vi "test_VISAFactory_InitializeMeasurementLinkSessionWithAttachAndDetach_RemoteSessionAttachedAndDetached.vi"(8 "error in":errorcluster) -> (0 "error out":errorcluster, 2 "result":string, 3 "pass":bool)   [LabVIEW 2020, in "MeasurementServerTests.lvlib"]
uses:
  MeasurementServerTests.lvlib
  Runtime/Sessions/Instrument Sessions/ISession Factory/Initialize and Close Session Behavior.ctl
  Runtime/Sessions/Instrument Sessions/ISession Factory/ISession Factory.lvclass
  Runtime/Sessions/VISA Sessions/Session Factory/Session Factory.lvclass
  <vilib>/Instr/_visa.llb/VISA Open Access Mode.ctl
  <vilib>/NI-VISA/VISA gRPC Open Close Behavior.ctl
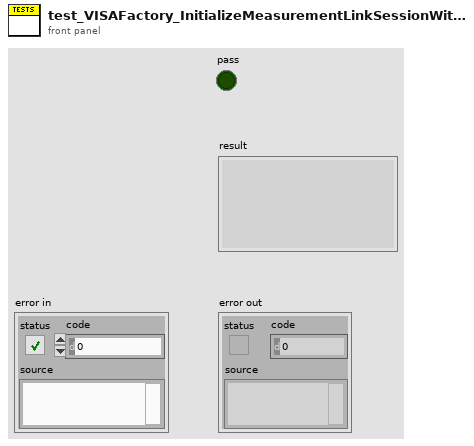
[diagram p1: front panel]
types:
  T1 = typedef "VISA gRPC Open Close Behavior.ctl" = enum16{"Auto", "Initialize and Close", "Attach and Detach", "Initialize and Detach", "Attach and Close"}
  T2 = typedef "VISA Open Access Mode.ctl" = u32
  T3 = typedef "Plug-In SDK Instrument Sessions.lvlib/ISession Factory.lvclass/Remote Connection Options.ctl" = cluster{"session name":string, "address":string, "port":u32}
  T4 = typedef "Plug-In SDK Instrument Sessions.lvlib/ISession Factory.lvclass/Initialize and Close Session Behavior.ctl" = enum16{"Initialize and Close", "Attach and Detach", "Initialize and Detach", "Attach and Close"}
  T5 = typedef "Plug-In SDK Instrument Sessions.lvlib/ISession Factory.lvclass/Session Initialization Parameters.ctl" = cluster{"resource name":string, "session name":string}
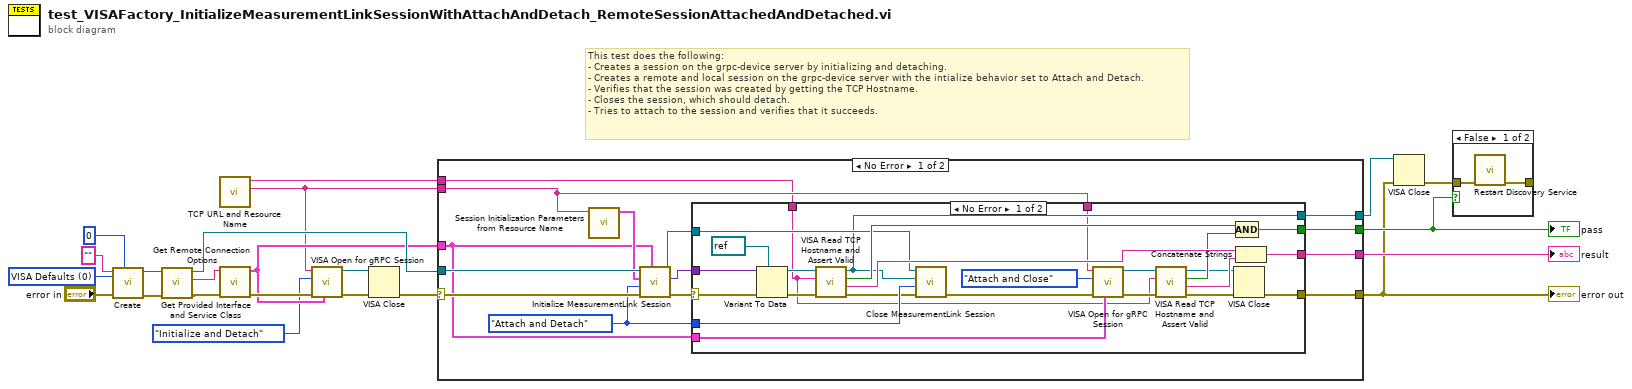
[diagram p0: block diagram]
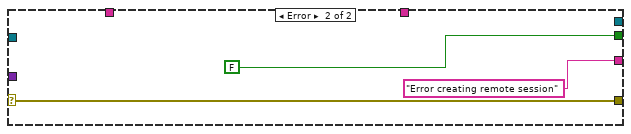
[diagram p2: hidden frame]
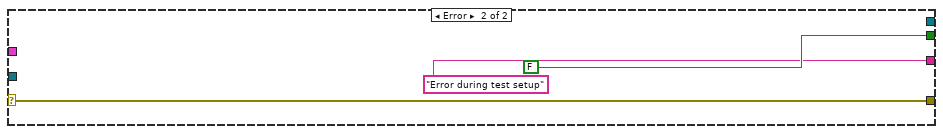
[diagram p3: hidden frame]
diagram:
  w9 = T2 0 items=["VISA Defaults"=0, "Exclusive Lock"=1, "Load Configured Settings"=4] ("access mode")
  # "This test does the following:\n- Creates a session on the grpc-device server by initializing and detaching.\n- Creates a remote and local session on the grpc-device server with the intialize behavior set to Attach and Detach.\n- Verifies that the session was created by getting the TCP Hostname.\n- Closes the session, which should detach.\n- Tries to attach to the session and verifies that it succeeds."
  n1 = call "Create.vi"("visa open timeout"=u32 0, "error in"="error in", "access mode"=w9, "instrument type id"="") -> ("error out"=w14:errorcluster, "session factory out"=w13:refnum<class "Session Factory.lvclass">)  [unwired: 6 in]
  n2 = call-dynamic "Get Provided Interface and Service Class.vi"("error in"=w14, "session factory in"=w13) -> ("error out"=w15:errorcluster, "provided interface"=w12:string, "session factory out"=w16:refnum<class "Session Factory.lvclass">)  [unwired: 6 in, 1 out]
  n3 = call "TCP URL and Resource Name.vi"() -> ("visa resource name"=w2:string, "url"=w1:string)  [unwired: 10 in]
  n4 = call "Get Remote Connection Options.vi"("error in"=w15, "provided interface"=w12) -> ("error out"=w8:errorcluster, "remote connection options"=w7:T3)  [unwired: 8 in]
  n5 = call <vilib>:"VISA Open for gRPC Session.vi"("gRPC Options"=w7, "error in (no error)"=w8, "open/close behavior"=VISA_gRPC_Open_Close_Behavior."Initialize and Detach" ("Open/Close Behavior"), "VISA resource name"=w2) -> ("error out"=w4:errorcluster, "VISA resource name out"=w3:refnum<visa-resource-name>)  [unwired: 6 in]
  n6 = VISA Close(VISA resource name=w3, error in (no error)=w4) -> (error out=w5:errorcluster)
  n7 = case shown="No Error" w5 {
    selector: w5 -> [w31 w65]
    tunnel: [w35 w65] -> w18
    tunnel: [w36 FALSE] -> w19
    tunnel: [w34 "Error during test setup" ("f")] -> w22
    tunnel: w7 -> [w25 _]
    tunnel: w16 -> [w30 _]
    tunnel: [w29 _] -> w21
    tunnel: w2 -> [w24 _]
    tunnel: w1 -> [w23 _]
    frame No Error {
      w26 = Initialize_and_Close_Session_Behavior."Attach and Detach" ("initialize and close session behavior")
      n8 = call "Session Initialization Parameters from Resource Name.vi"("resource name"=w24) -> ("session initialization parameters"=w28:T5)  [unwired: 10 in]
      n9 = call-dynamic "Initialize MeasurementLink Session.vi"("remote connection options"=w25, "error in"=w31, "initialize and close session behavior"=w26, "session initialization parameters"=w28, "session factory in"=w30) -> ("error out"=w32:errorcluster, "session out"=w33:variant, "session factory out"=w27:refnum<class "Session Factory.lvclass">)  [unwired: 4 in]
      n10 = case shown="No Error" w32 {
        selector: w32 -> [w60 w63]
        tunnel: [w56 FALSE] -> w36
        tunnel: [w46 w63] -> w35
        tunnel: [w54 "Error creating remote session"] -> w34
        tunnel: w33 -> [w61 _]
        tunnel: [w51 _] -> w29
        tunnel: w27 -> [w52 _]
        tunnel: w26 -> [w50 _]
        tunnel: w24 -> [w48 _]
        tunnel: w25 -> [w45 _]
        tunnel: w23 -> [w37 _]
        frame No Error {
          n11 = Variant To Data(error in=w60, type=refnum<visa-resource-name> refnum ("VISA resource name out"), Variant=w61) -> (data=w57:refnum<visa-resource-name>, error out=w58:errorcluster)
          n12 = call "VISA Read TCP Hostname and Assert Valid.vi"("error in"=w58, "expected hostname"=w37, "visa refnum in"=w57) -> ("error out"=w44:errorcluster, "result"=w53:string, "pass?"=w55:bool, "visa refnum out"=w51:refnum<visa-resource-name>)  [unwired: 5 in]
          n13 = call-dynamic "Close MeasurementLink Session.vi"("error in"=w44, "initialize and close session behavior"=w50, "session in"=w51, "session factory in"=w52) -> ("error out"=w49:errorcluster)  [unwired: 7 in]
          n14 = call <vilib>:"VISA Open for gRPC Session.vi"("gRPC Options"=w45, "error in (no error)"=w49, "open/close behavior"=VISA_gRPC_Open_Close_Behavior."Attach and Close" ("Open/Close Behavior"), "VISA resource name"=w48) -> ("error out"=w43:errorcluster, "VISA resource name out"=w39:refnum<visa-resource-name>)  [unwired: 6 in]
          n15 = call "VISA Read TCP Hostname and Assert Valid.vi"("error in"=w43, "expected hostname"=w37, "visa refnum in"=w39) -> ("error out"=w42:errorcluster, "result"=w41:string, "pass?"=w40:bool, "visa refnum out"=w38:refnum<visa-resource-name>)  [unwired: 5 in]
          n16 = VISA Close(VISA resource name=w38, error in (no error)=w42) -> (error out=w46:errorcluster)
          n17 = Compound Arithmetic op=AND(w55, w40) -> (w56:bool)
          n18 = Concatenate Strings(w53, w41) -> (w54:string)
        }
        frame Error {
        }
      }
    }
    frame Error {
    }
  }
  "error out" <- w18
  "pass" <- w19
  "result" <- w22
  n19 = VISA Close(VISA resource name=w21, error in (no error)=w18) -> (error out=w20:errorcluster)
  n20 = case shown="False" w19 {
    tunnel: w20 -> [w69 _]
    tunnel: [w68 _] -> _
    frame False {
      n21 = call "Restart Discovery Service.vi"("error in"=w69) -> ("error out"=w68:errorcluster)  [unwired: 10 in]
    }
    frame True {
    }
  }
